vi "Robot.vi"(1 "error in":errorcluster, 2 "Type":enum16{"Mini45", "Simulation", "Joystick"}(ring)=enum."Simulation") -> (0 "error out":errorcluster)   [LabVIEW 2017]
uses:
  <vilib>/Analysis/Matrix/Datatypes/RealMatrix.ctl
  Control/Motor Position.ctl
  Control/Constants.ctl
  Control/Platform Vectors.ctl
  Control/Force Torque Vector.ctl
  Control/RPY.ctl
  <vilib>/Analysis/baseanly.llb/A x Vector.vi
  <vilib>/Analysis/baseanly.llb/Mean (DBL).vi
  <vilib>/Analysis/_algsub.llb/Real Vector Norm.vi
  <vilib>/Analysis/baseanly.llb/Real A x B.vi
  <vilib>/DAQmx/read.llb/DAQmx Read (Analog 2D DBL NChan NSamp).vi
  <vilib>/Analysis/baseanly.llb/Outer Product.vi
  <vilib>/Analysis/baseanly.llb/Real Outer Product.vi
  <vilib>/robotics/Kinematics/Create Lie Group Matrix.vi
  <vilib>/Analysis/7linalg.llb/Create Special Real Matrix.vi
  <vilib>/Analysis/Matrix/Numeric/Multiply/Multiply.vi
  <vilib>/Analysis/Matrix/Numeric/Multiply/Multiply - RM,R.vi
  <vilib>/Analysis/Matrix/Numeric/Multiply/Multiply - R,RM.vi
  <vilib>/Analysis/Matrix/Numeric/Add/Add.vi
  <vilib>/Analysis/Matrix/Numeric/Add/Add - RM,RM.vi
  <vilib>/Analysis/3filter.llb/Butterworth Filter (DBL).vi
  Global.vi
  <vilib>/Utility/inputDevices.llb/joystickAcquire.vi
  <vilib>/DAQmx/create/channels.llb/DAQmx Create Channel (AI-Voltage-Basic).vi
  <vilib>/DAQmx/configure/timing.llb/DAQmx Timing (Sample Clock).vi
  <vilib>/DAQmx/miscellaneous.llb/DAQmx Fill In Error Info.vi
  <vilib>/Analysis/NI_AALBase.lvlib
  <vilib>/robotics/Kinematics/NI_Kinematics.lvlib
  <vilib>/Analysis/NI_AALPro.lvlib
  <vilib>/ptbypt/NI_PtbyPt.lvlib
  <vilib>/Analysis/Matrix/NI_Matrix.lvlib
panel:
  in  "low cutoff freq: fl":dbl=0.1 format="%0.4f"
  in  "sampling freq: fs":dbl=100.0 format="%0.2f"
  in  "rate":dbl=1000.0 format="%#_13g"
  in  "eta3":dbl=240.0
  in  "eta2":dbl=120.0
  in  "eta1":dbl
  in  "gamma2":dbl=72.0
  in  "gamma1":dbl=90.0
  in  "alpha2":dbl=90.0
  in  "alpha1":dbl=90.0
  in  "radius":dbl=0.1
  in  "Calibration Matrix":T1=[[0.70287, 0.28046, -1.06379, -47.58271, -1.64459, 46.90249], [-0.12905, 55.12684, -1.23322, -27.09022, 0.94146, -27.44249], [69.23154, 1.17633, 67.18151, 0.05352, 69.14468, -0.82584], [0.02366, 0.38743, -1.10802, -0.19684, 1.1351, -0.20033], [1.26658, 0.02633, -0.60731, 0.32903, -0.6386, -0.32248], [0.02624, -0.70869, -0.00313, -0.69424, -0.02408, -0.68399]]
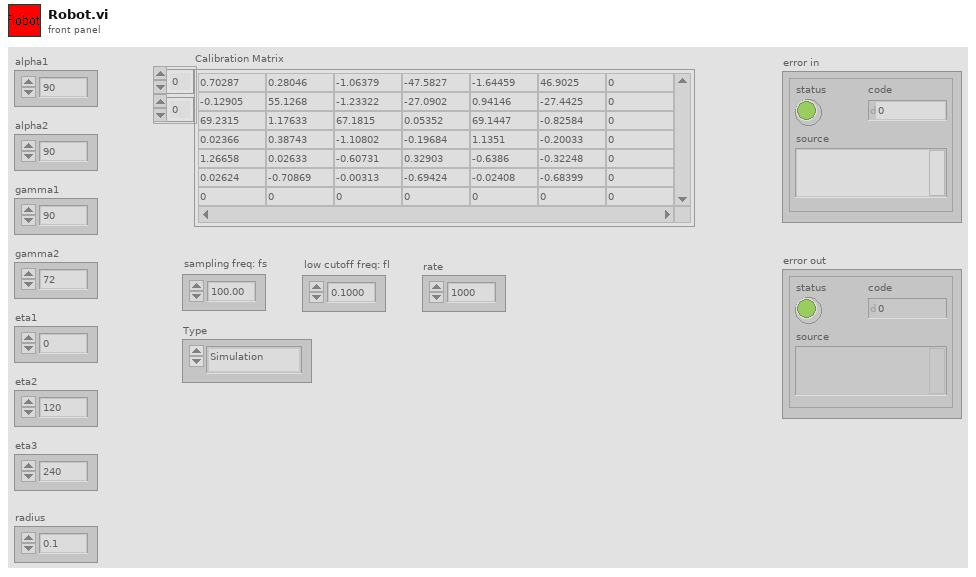
[diagram p1: front panel]
types:
  T1 = typedef "NI_Matrix.lvlib/RealMatrix.ctl" = dbl[][]
  T2 = typedef "Motor Position.ctl" = cluster{"theta1":dbl, "theta2":dbl, "theta3":dbl}
  T3 = typedef "Platform Vectors.ctl" = cluster{"v1":dbl[], "v2":dbl[], "v3":dbl[]}
  T4 = typedef "Constants.ctl" = cluster{"alpha1":dbl, "alpha2":dbl, "beta1":dbl, "beta2":dbl, "gamma1":dbl, "gamma2":dbl, "eta1":dbl, "eta2":dbl, "eta3":dbl}
  T5 = typedef "Force Torque Vector.ctl" = cluster{"Fx":dbl, "Fy":dbl, "Tz":dbl}
  T6 = typedef "RPY.ctl" = cluster{"roll":dbl, "pitch":dbl, "yaw":dbl}
  T7 = cluster{"X axis":i32, "Y axis":i32, "Z axis":i32, "X axis rotation":i32, "Y axis rotation":i32, "Z axis rotation":i32, "U axis":i32, "V axis":i32}
  T8 = typedef "Damping.ctl" = cluster{"Cx":dbl, "Cy":dbl, "Cz":dbl}
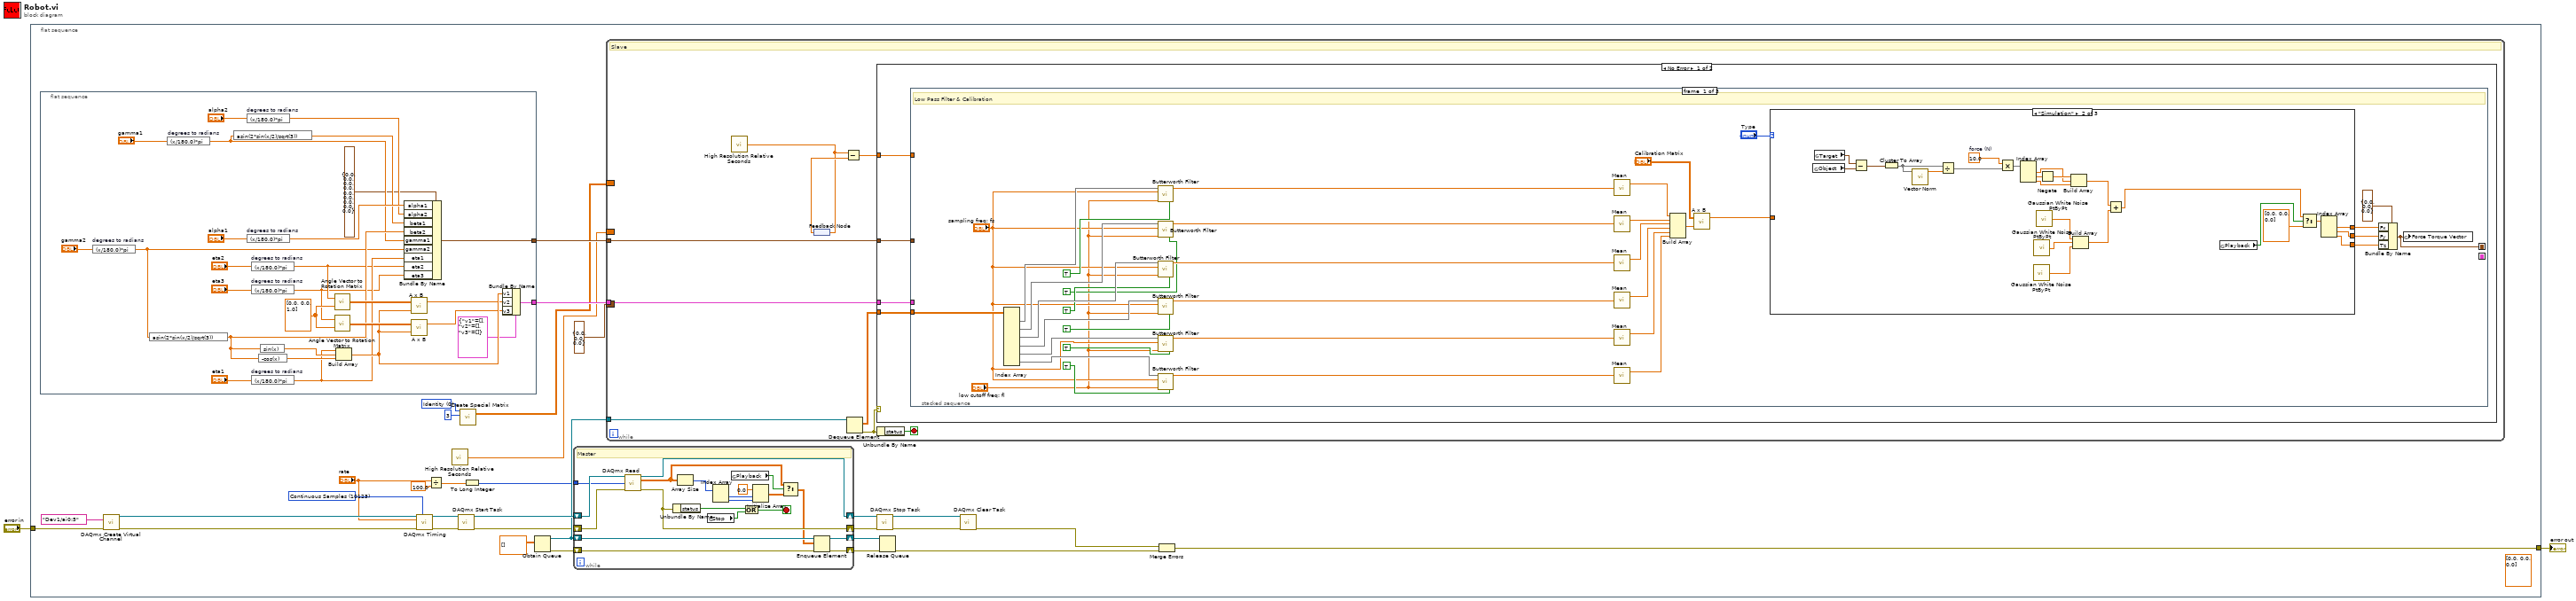
[diagram p0: block diagram]
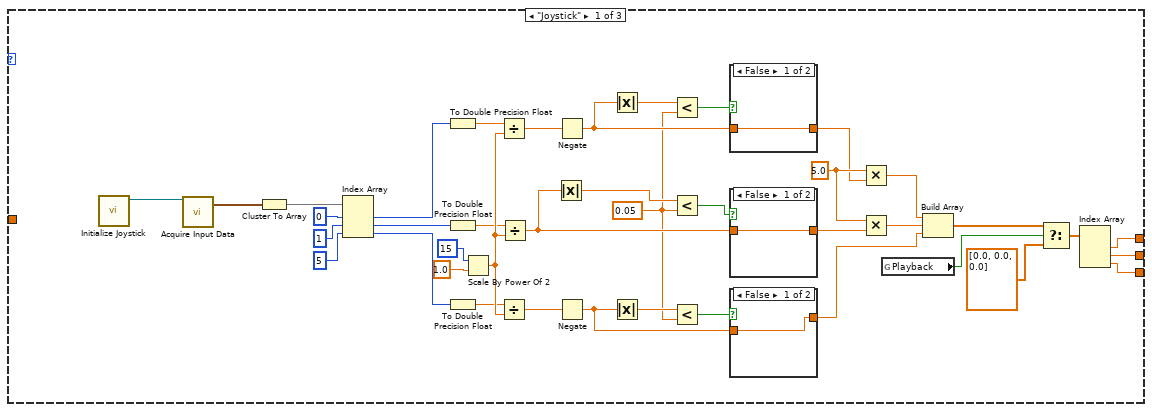
[diagram p2: hidden frame]
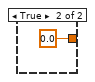
[diagram p3: hidden frame]
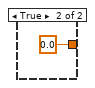
[diagram p4: hidden frame]
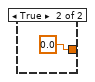
[diagram p5: hidden frame]
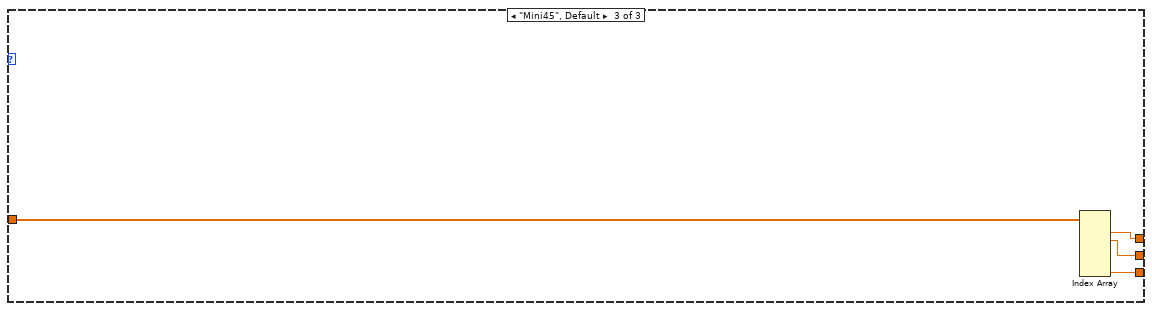
[diagram p6: hidden frame]
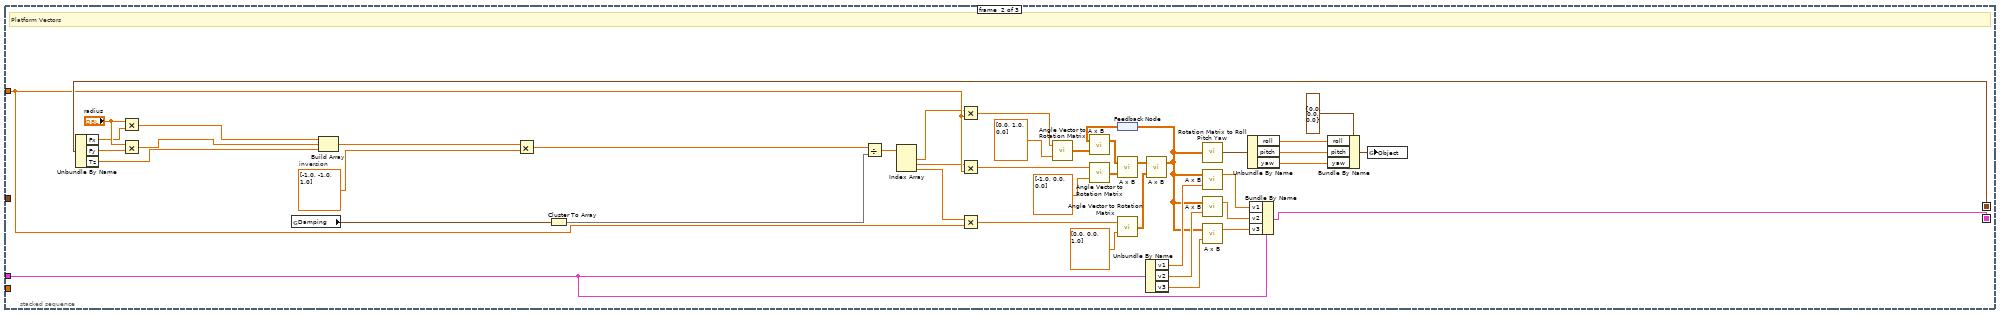
[diagram p7: hidden frame]
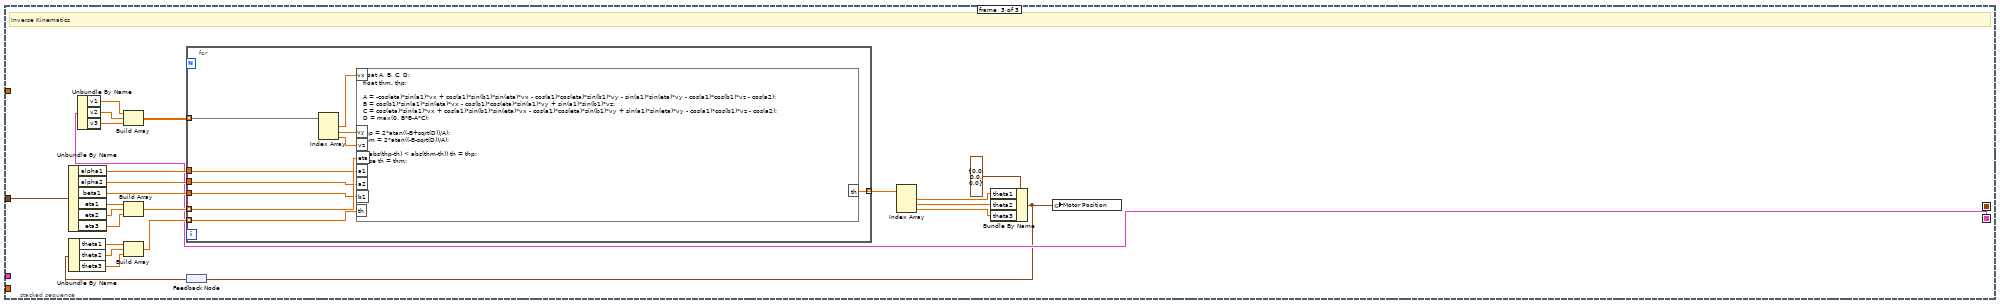
[diagram p8: hidden frame]
diagram:
  n1 = flat-sequence {
    tunnel: "error in" -> [w5]
    tunnel: [w3] -> w1
    frame #0 {
      w16 = 0 items=["Identity", "Diagonal", "Toeplitz", "Vandermonde", "Companion", "Hankel", "Hadamard", "Wilkinson", "Hilbert", "Inverse Hilbert", "Rosser", "Pascal"] ("matrix type")
      (unwired) dbl[] [0.0, 0.0, 0.0]
      w22 = 10123 items=["Finite Samples"=10178, "Continuous Samples"=10123, "Hardware Timed Single Point"=12522] ("sample mode")
      n2 = flat-sequence {
        tunnel: [w62] -> w34
        tunnel: [w61] -> w33
        frame #0 {
          w49 = dbl[] [0.0, 0.0, 1.0] ("vector")
          n3 = expression code="(x/180.0)*pi" "degrees to radians"("gamma2") -> (w43:dbl)
          n4 = expression code="asin(2*sin(x/2)/sqrt(3))"(w43) -> (w45:dbl)
          n5 = expression code="(x/180.0)*pi" "degrees to radians"("gamma1") -> (w44:dbl)
          n6 = expression code="asin(2*sin(x/2)/sqrt(3))"(w44) -> (w56:dbl)
          n7 = expression code="(x/180.0)*pi" "degrees to radians"("alpha2") -> (w57:dbl)
          n8 = expression code="(x/180.0)*pi" "degrees to radians"("alpha1") -> (w59:dbl)
          n9 = expression code="(x/180.0)*pi" "degrees to radians"("eta2") -> (w38:dbl)
          n10 = expression code="(x/180.0)*pi" "degrees to radians"("eta3") -> (w37:dbl)
          n11 = expression code="(x/180.0)*pi" "degrees to radians"("eta1") -> (w39:dbl)
          n12 = expression code="-cos(x)"(w45) -> (w51:dbl)
          n13 = expression code="sin(x)"(w45) -> (w50:dbl)
          n14 = call <vilib>:"Angle Vector to Rotation Matrix.vi"("vector"=w49, "angle"=w38) -> ("rotation matrix"=w52:T1)
          n15 = call <vilib>:"Angle Vector to Rotation Matrix.vi"("vector"=w49, "angle"=w37) -> ("rotation matrix"=w53:T1)
          n16 = Build Array(w39, w50, w51) -> (w48:dbl[])
          n17 = Bundle By Name(cluster=T4 {"alpha1"=0.0, "alpha2"=0.0, "beta1"=0.0, "beta2"=0.0, "gamma1"=0.0, "gamma2"=0.0, "eta1"=0.0, "eta2"=0.0, "eta3"=0.0} ("Constants"), "alpha1"=w59, "alpha2"=w57, "beta1"=w56, "beta2"=w45, "gamma1"=w44, "gamma2"=w43, "eta1"=w39, "eta2"=w38, "eta3"=w37) -> (w61:T4)
          n18 = call-poly <vilib>:"A x B.vi"("Vector"=w48, "A"=w52) -> ("A x Vector"=w47:dbl[])  [unwired: 1 out]
          n19 = call-poly <vilib>:"A x B.vi"("Vector"=w48, "A"=w53) -> ("A x Vector"=w46:dbl[])  [unwired: 1 out]
          n20 = Bundle By Name(cluster=T3 {"v1"=[], "v2"=[], "v3"=[]} ("Platform Vectors"), "v1"=w48, "v2"=w47, "v3"=w46) -> (w62:T3)
        }
      }
      n21 = call-poly <vilib>:"DAQmx Create Virtual Channel.vi"("physical channels"=tag "Dev1/ai0:5", "error in"=w5) -> ("task out"=w31:refnum<k21>, "error out"=w30:errorcluster)  [unwired: 12 in]
      n22 = call-poly <vilib>:"DAQmx Timing.vi"("task/channels in"=w31, "sample mode"=w22, "rate"="rate", "error in"=w30) -> ("task out"=w28:refnum<k21>, "error out"=w29:errorcluster)  [unwired: 10 in]
      n23 = Divide(x="rate", y=100.0) -> (x/y=w6:dbl)
      n24 = call <vilib>:"High Resolution Relative Seconds.vi"() -> ("relative seconds"=w7:dbl)
      n25 = call <vilib>:"DAQmx Start Task.vi"("task/channels in"=w28, "error in"=w29) -> ("task out"=w27:refnum<k21>, "error out"=w4:errorcluster)  [unwired: 12 in]
      n26 = call-poly <vilib>:"Create Special Matrix.vi"("matrix type"=w16, "matrix size"=3) -> ("Special Matrix"=w14:T1)  [unwired: 3 in, 1 out]
      n27 = To Long Integer(number=w6) -> (32bit integer=w9:i32)
      n28 = Obtain Queue(element data type=dbl[][] [] ("data")) -> (queue out=w12:refnum<queue>, error out=w21:errorcluster)  [unwired: 4 in, 1 out]
      n29 = while {
        shift-right: [w278] -> w19
        shift-left: w12 -> [w279]
        shift-right: [w275] -> w18
        shift-left: w21 -> [w277]
        shift-right: [w282] -> w26
        shift-left: w27 -> [w283]
        shift-right: [w280] -> w24
        shift-left: w4 -> [w281]
        tunnel: w9 -> [w273]
        stop <- w274 stop-if-true
        # "Master"
        n30 = call-poly <vilib>:"DAQmx Read.vi"("task/channels in"=w283, "number of samples per channel"=w273, "error in"=w281) -> ("task out"=w282:refnum<k21>, "data"=w269:dbl[][], "error out"=w280:errorcluster)  [unwired: 10 in]
        n31 = Unbundle By Name(w280) -> ("status"=w276:bool)
        n32 = Array Size(array=w269) -> (size(s)=w268:i32[])
        n33 = global read "Global.vi" "Stop"() -> (w272:bool)
        n34 = Index Array(array=w268) -> (element #1=w267:i32, element #2=w266:i32)  [unwired: 2 in]
        n35 = global read "Global.vi" "Playback"() -> (w271:bool)
        n36 = Compound Arithmetic op=OR(w276, w272) -> (w274:bool)
        n37 = Initialize Array(0.0 ("element"), w267, w266) -> (w264:dbl[][])
        n38 = Select(t=w269, s=w271, f=w264) -> (s? t:f=w270:dbl[][])
        n39 = Enqueue Element(queue=w279, element=w270, error in (no error)=w277) -> (queue out=w278:refnum<queue>, error out=w275:errorcluster)  [unwired: 1 in, 1 out]
      }
      n40 = while {
        tunnel: w12 -> [w71]
        border: w14 -> [_]
        tunnel: w33 -> [w69]
        border: T2 {"theta1"=0.0, "theta2"=0.0, "theta3"=0.0} ("Motor Position") -> [_]
        border: w7 -> [_]
        tunnel: w34 -> [w70]
        stop <- w63 stop-if-true
        # "Slave"
        n41 = call <vilib>:"High Resolution Relative Seconds.vi"() -> ("relative seconds"=w65:dbl)
        n42 = feedback-in #1(w65) -> ()
        n43 = feedback #1() -> (w66:dbl)
        n44 = Subtract(x=w65, y=w66) -> (x-y=w64:dbl)
        n45 = Dequeue Element(queue=w71) -> (element=w67:dbl[][], error out=w68:errorcluster)  [unwired: 2 in, 2 out]
        n46 = case shown="No Error" w68 {
          tunnel: w70 -> [w75 _]
          tunnel: w69 -> [w74 _]
          tunnel: w67 -> [w73 _]
          tunnel: w64 -> [w72 _]
          frame No Error {
            n47 = stacked-sequence {
              seq-local: [w76 _ _] -> [_ w219 _]
              seq-local: [_ w205 _] -> [_ _ w232]
              tunnel: w75 -> [_ w208 _]
              tunnel: w74 -> [_ _ w249]
              tunnel: w72 -> [_ w204 _]
              tunnel: w73 -> [w87 _ _]
              frame #0 {
                # "Low Pass Filter & Calibration"
                n48 = Index Array(array=w87) -> (element #1=w98:dbl[], element #2=w97:dbl[], element #3=w96:dbl[], element #4=w95:dbl[], element #5=w94:dbl[], element #6=w93:dbl[])  [unwired: 12 in]
                n49 = call-poly <vilib>:"Butterworth Filter.vi"("init/cont (init:F)"=TRUE, "low cutoff freq: fl"="low cutoff freq: fl", "sampling freq: fs"="sampling freq: fs", "X"=w98) -> ("Filtered X"=w99:dbl[])  [unwired: 4 in, 1 out]
                n50 = call-poly <vilib>:"Butterworth Filter.vi"("init/cont (init:F)"=TRUE, "low cutoff freq: fl"="low cutoff freq: fl", "sampling freq: fs"="sampling freq: fs", "X"=w97) -> ("Filtered X"=w101:dbl[])  [unwired: 4 in, 1 out]
                n51 = call-poly <vilib>:"Butterworth Filter.vi"("init/cont (init:F)"=TRUE, "low cutoff freq: fl"="low cutoff freq: fl", "sampling freq: fs"="sampling freq: fs", "X"=w96) -> ("Filtered X"=w103:dbl[])  [unwired: 4 in, 1 out]
                n52 = call-poly <vilib>:"Butterworth Filter.vi"("init/cont (init:F)"=TRUE, "low cutoff freq: fl"="low cutoff freq: fl", "sampling freq: fs"="sampling freq: fs", "X"=w95) -> ("Filtered X"=w104:dbl[])  [unwired: 4 in, 1 out]
                n53 = call-poly <vilib>:"Butterworth Filter.vi"("init/cont (init:F)"=TRUE, "low cutoff freq: fl"="low cutoff freq: fl", "sampling freq: fs"="sampling freq: fs", "X"=w94) -> ("Filtered X"=w105:dbl[])  [unwired: 4 in, 1 out]
                n54 = call-poly <vilib>:"Butterworth Filter.vi"("init/cont (init:F)"=TRUE, "low cutoff freq: fl"="low cutoff freq: fl", "sampling freq: fs"="sampling freq: fs", "X"=w93) -> ("Filtered X"=w109:dbl[])  [unwired: 4 in, 1 out]
                n55 = call-poly <vilib>:"Mean.vi"("X"=w99) -> ("mean"=w100:dbl)  [unwired: 1 out]
                n56 = call-poly <vilib>:"Mean.vi"("X"=w101) -> ("mean"=w102:dbl)  [unwired: 1 out]
                n57 = call-poly <vilib>:"Mean.vi"("X"=w103) -> ("mean"=w106:dbl)  [unwired: 1 out]
                n58 = call-poly <vilib>:"Mean.vi"("X"=w104) -> ("mean"=w107:dbl)  [unwired: 1 out]
                n59 = call-poly <vilib>:"Mean.vi"("X"=w105) -> ("mean"=w108:dbl)  [unwired: 1 out]
                n60 = call-poly <vilib>:"Mean.vi"("X"=w109) -> ("mean"=w110:dbl)  [unwired: 1 out]
                n61 = Build Array(w100, w102, w106, w107, w108, w110) -> (w85:dbl[])
                n62 = call-poly <vilib>:"A x B.vi"("Vector"=w85, "A"="Calibration Matrix") -> ("A x Vector"=w81:dbl[])  [unwired: 1 out]
                n63 = case shown="\"Simulation\"" "Type" {
                  tunnel: w81 -> [_ _ w185]
                  tunnel: [w115 w181 w184] -> w79
                  tunnel: [w114 w180 w183] -> w78
                  tunnel: [w113 w179 w182] -> w77
                  frame "Joystick" {
                    w124 = 5.0 ("element")
                    w131 = 0.05 ("y")
                    n64 = call <vilib>:"Initialize Joystick.vi"() -> ("device ID"=w144:refnum<k1>)  [unwired: 10 in, 1 out]
                    n65 = call-poly <vilib>:"Acquire Input Data.vi"("device ID"=w144) -> ("axis info"=w151:T7)  [unwired: 14 in, 4 out]
                    n66 = Cluster To Array(cluster=w151) -> (array=w147:i32[])
                    n67 = Index Array(array=w147, index #1=0 ("index"), index #2=1 ("index"), index #3=5 ("index")) -> (element #1=w130:i32, element #2=w128:i32, element #3=w126:i32)
                    n68 = To Double Precision Float(number=w130) -> (double precision float=w129:dbl)
                    n69 = To Double Precision Float(number=w128) -> (double precision float=w127:dbl)
                    n70 = To Double Precision Float(number=w126) -> (double precision float=w125:dbl)
                    n71 = Scale By Power Of 2(n=i16 15, x=1.0) -> (x*2^n=w139:dbl)
                    n72 = Divide(x=w129, y=w139) -> (x/y=w143:dbl)
                    n73 = Divide(x=w125, y=w139) -> (x/y=w132:dbl)
                    n74 = Divide(x=w127, y=w139) -> (x/y=w134:dbl)
                    n75 = Absolute Value(x=w134) -> (abs(x)=w141:dbl)
                    n76 = Negate(x=w143) -> (-x=w135:dbl)
                    n77 = Negate(x=w132) -> (-x=w133:dbl)
                    n78 = Absolute Value(x=w135) -> (abs(x)=w142:dbl)
                    n79 = Absolute Value(x=w133) -> (abs(x)=w140:dbl)
                    n80 = Less?(x=w142, y=w131) -> (x < y?=w138:bool)
                    n81 = Less?(x=w141, y=w131) -> (x < y?=w137:bool)
                    n82 = Less?(x=w140, y=w131) -> (x < y?=w136:bool)
                    n83 = case shown="False" w138 {
                      tunnel: [w156 0.0] -> w123
                      tunnel: w135 -> [w156 _]
                      frame False {
                      }
                      frame True {
                      }
                    }
                    n84 = case shown="False" w137 {
                      tunnel: [w154 0.0] -> w122
                      tunnel: w134 -> [w154 _]
                      frame False {
                      }
                      frame True {
                      }
                    }
                    n85 = case shown="False" w136 {
                      tunnel: [w152 0.0] -> w118
                      tunnel: w133 -> [w152 _]
                      frame False {
                      }
                      frame True {
                      }
                    }
                    n86 = Multiply(x=w124, y=w123) -> (x*y=w120:dbl)
                    n87 = Multiply(x=w124, y=w122) -> (x*y=w119:dbl)
                    n88 = global read "Global.vi" "Playback"() -> (w121:bool)
                    n89 = Build Array(w120, w119, w118) -> (w117:dbl[])
                    n90 = Select(t=w117, s=w121, f=dbl[] [0.0, 0.0, 0.0]) -> (s? t:f=w116:dbl[])
                    n91 = Index Array(array=w116) -> (element #1=w115:dbl, element #2=w114:dbl, element #3=w113:dbl)  [unwired: 3 in]
                  }
                  frame "Simulation" {
                    w171 = 10.0  # force (N)
                    n92 = global read "Global.vi" "Object"() -> (w169:T6)
                    n93 = global read "Global.vi" "Target"() -> (w170:T6)
                    n94 = Subtract(x=w170, y=w169) -> (x-y=w175:T6)
                    n95 = Cluster To Array(cluster=w175) -> (array=w174:dbl[])
                    n96 = call-poly <vilib>:"Vector Norm.vi"("Input Vector"=w174) -> ("norm"=w173:dbl)  [unwired: 9 in, 1 out]
                    n97 = Divide(x=w174, y=w173) -> (x/y=w172:dbl[])
                    n98 = Multiply(x=w171, y=w172) -> (x*y=w166:dbl[])
                    n99 = Index Array(array=w166) -> (element #1=w165:dbl, element #2=w168:dbl, element #3=w164:dbl)  [unwired: 3 in]
                    n100 = call <vilib>:"Gaussian White Noise PtByPt.vi"() -> ("Gaussian white noise"=w161:dbl)  [unwired: 3 in]
                    n101 = call <vilib>:"Gaussian White Noise PtByPt.vi"() -> ("Gaussian white noise"=w162:dbl)  [unwired: 3 in]
                    n102 = call <vilib>:"Gaussian White Noise PtByPt.vi"() -> ("Gaussian white noise"=w163:dbl)  [unwired: 3 in]
                    n103 = Negate(x=w168) -> (-x=w167:dbl)
                    n104 = Build Array(w167, w165, w164) -> (w160:dbl[])
                    n105 = Build Array(w163, w162, w161) -> (w159:dbl[])
                    n106 = Add(x=w160, y=w159) -> (x+y=w158:dbl[])
                    n107 = global read "Global.vi" "Playback"() -> (w176:bool)
                    n108 = Select(t=w158, s=w176, f=dbl[] [0.0, 0.0, 0.0]) -> (s? t:f=w178:dbl[])
                    n109 = Index Array(array=w178) -> (element #1=w181:dbl, element #2=w180:dbl, element #3=w179:dbl)  [unwired: 3 in]
                  }
                  frame "Mini45", Default {
                    n110 = Index Array(array=w185) -> (element #1=w184:dbl, element #2=w183:dbl, element #6=w182:dbl)  [unwired: 6 in, 3 out]
                  }
                }
                n111 = Bundle By Name(cluster=T5 {"Fx"=0.0, "Fy"=0.0, "Tz"=0.0} ("Force Torque Vector"), "Fx"=w79, "Fy"=w78, "Tz"=w77) -> (w76:T5)
                n112 = global write "Global.vi" "Force Torque Vector"(w76) -> ()
              }
              frame #1 {
                w206 = dbl[] [-1.0, -1.0, 1.0]  # inversion
                # "Platform Vectors"
                n113 = Unbundle By Name(w219) -> ("Fx"=w217:dbl, "Fy"=w216:dbl, "Tz"=w213:dbl)
                n114 = Multiply(x="radius", y=w217) -> (x*y=w215:dbl)
                n115 = Multiply(x="radius", y=w216) -> (x*y=w214:dbl)
                n116 = global read "Global.vi" "Damping"() -> (w191:T8)
                n117 = Build Array(w215, w214, w213) -> (w207:dbl[])
                n118 = Multiply(x=w207, y=w206) -> (x*y=w192:dbl[])
                n119 = Cluster To Array(cluster=w191) -> (array=w190:dbl[])
                n120 = Divide(x=w192, y=w190) -> (x/y=w189:dbl[])
                n121 = Index Array(array=w189) -> (element #1=w188:dbl, element #2=w187:dbl, element #3=w186:dbl)  [unwired: 3 in]
                n122 = Multiply(x=w188, y=w204) -> (x*y=w229:dbl)
                n123 = Multiply(x=w187, y=w204) -> (x*y=w228:dbl)
                n124 = Multiply(x=w186, y=w204) -> (x*y=w203:dbl)
                n125 = call <vilib>:"Angle Vector to Rotation Matrix.vi"("vector"=dbl[] [0.0, 1.0, 0.0], "angle"=w229) -> ("rotation matrix"=w224:T1)
                n126 = call <vilib>:"Angle Vector to Rotation Matrix.vi"("vector"=dbl[] [-1.0, 0.0, 0.0], "angle"=w228) -> ("rotation matrix"=w222:T1)
                n127 = feedback #2() -> (w212:T1)
                n128 = call-poly <vilib>:"A x B.vi"("B"=w224, "A"=w212) -> ("A x B"=w223:T1)  [unwired: 1 out]
                n129 = call-poly <vilib>:"A x B.vi"("B"=w222, "A"=w223) -> ("A x B"=w221:T1)  [unwired: 1 out]
                n130 = call <vilib>:"Angle Vector to Rotation Matrix.vi"("vector"=dbl[] [0.0, 0.0, 1.0], "angle"=w203) -> ("rotation matrix"=w220:T1)
                n131 = Unbundle By Name(w208) -> ("v1"=w211:dbl[], "v2"=w210:dbl[], "v3"=w209:dbl[])
                n132 = call-poly <vilib>:"A x B.vi"("B"=w220, "A"=w221) -> ("A x B"=w199:T1)  [unwired: 1 out]
                n133 = feedback-in #2(w199) -> ()
                n134 = call <vilib>:"Rotation Matrix to Roll Pitch Yaw.vi"("rotation matrix"=w199) -> ("angles"=w197:cluster{"roll":dbl, "pitch":dbl, "yaw":dbl})
                n135 = call-poly <vilib>:"A x B.vi"("Vector"=w211, "A"=w199) -> ("A x Vector"=w202:dbl[])  [unwired: 1 out]
                n136 = call-poly <vilib>:"A x B.vi"("Vector"=w210, "A"=w199) -> ("A x Vector"=w201:dbl[])  [unwired: 1 out]
                n137 = call-poly <vilib>:"A x B.vi"("Vector"=w209, "A"=w199) -> ("A x Vector"=w200:dbl[])  [unwired: 1 out]
                n138 = Unbundle By Name(w197) -> ("roll"=w196:dbl, "pitch"=w195:dbl, "yaw"=w194:dbl)
                n139 = Bundle By Name(cluster=w208, "v1"=w202, "v2"=w201, "v3"=w200) -> (w205:T3)
                n140 = Bundle By Name(cluster=T6 {"roll"=0.0, "pitch"=0.0, "yaw"=0.0} ("RPY"), "roll"=w196, "pitch"=w195, "yaw"=w194) -> (w193:T6)
                n141 = global write "Global.vi" "Object"(w193) -> ()
              }
              frame #2 {
                # "Inverse Kinematics"
                n142 = Unbundle By Name(w249) -> ("alpha1"=w244:dbl, "alpha2"=w243:dbl, "beta1"=w242:dbl, "eta1"=w248:dbl, "eta2"=w247:dbl, "eta3"=w246:dbl)
                n143 = Unbundle By Name(w232) -> ("v1"=w253:dbl[], "v2"=w252:dbl[], "v3"=w251:dbl[])
                n144 = Build Array(w253, w252, w251) -> (w250:dbl[][])
                n145 = Build Array(w248, w247, w246) -> (w245:dbl[])
                n146 = feedback #3() -> (w237:T2)
                n147 = Unbundle By Name(w237) -> ("theta1"=w236:dbl, "theta2"=w235:dbl, "theta3"=w234:dbl)
                n148 = Build Array(w236, w235, w234) -> (w233:dbl[])
                n149 = for {
                  tunnel: w250 -> [w263] mode=indexing
                  tunnel: w245 -> [w259] mode=indexing
                  tunnel: w244 -> [w258]
                  tunnel: w243 -> [w257]
                  tunnel: w242 -> [w256]
                  tunnel: [w255] -> w241 mode=indexing
                  tunnel: w233 -> [w254] mode=indexing
                  n150 = Index Array(array=w263) -> (element #1=w262:dbl, element #2=w261:dbl, element #3=w260:dbl)  [unwired: 3 in]
                  n151 = formula code="float A, B, C, D;\nfloat thm, thp;\n\nA = -cos(eta)*sin(a1)*vx + cos(a1)*sin(b1)*sin(eta)*vx - cos(a1)*cos(eta)*sin(b1)*vy - sin(a1)*sin(eta)*vy - cos(a1)*cos(b1)*vz - cos(a2);\nB = cos(b1)*sin(a1)*sin(eta)*vx - cos(b1)*cos(eta)*sin(a1)*vy + sin(a1)*sin(b1)*vz;\nC = cos(eta)*sin(a1)*vx + cos(a1)*sin(b1)*sin(eta)*vx - cos(a1)*cos(eta)*sin(b1)*vy + sin(a1)*sin(eta)*vy - cos(a1)*cos(b1)*vz - cos(a2);\nD = max(0, B*B-A*C);\n\nthp = 2*atan((-B+sqrt(D))/A); \nthm = 2*atan((-B-sqrt(D))/A); \n\nif(abs(thp-th) < abs(thm-th)) th = thp;\nelse th = thm;"("vx"=w262, "vy"=w261, "vz"=w260, "eta"=w259, "a1"=w258, "b1"=w256, "a2"=w257, "th"=w254) -> ("th"=w255:dbl)
                }
                n152 = Index Array(array=w241) -> (element #1=w240:dbl, element #2=w239:dbl, element #3=w238:dbl)  [unwired: 3 in]
                n153 = Bundle By Name(cluster=T2 {"theta1"=0.0, "theta2"=0.0, "theta3"=0.0} ("Motor Position"), "theta1"=w240, "theta2"=w239, "theta3"=w238) -> (w230:T2)
                n154 = feedback-in #3(w230) -> ()
                n155 = global write "Global.vi" "Motor Position"(w230) -> ()
              }
            }
          }
          frame Error {
          }
        }
        n156 = Unbundle By Name(w68) -> ("status"=w63:bool)
      }
      n157 = call <vilib>:"DAQmx Stop Task.vi"("task/channels in"=w26, "error in"=w24) -> ("task out"=w25:refnum<k21>, "error out"=w23:errorcluster)  [unwired: 12 in]
      n158 = Release Queue(queue=w19, error in (no error)=w18) -> (error out=w17:errorcluster)  [unwired: 1 in, 2 out]
      n159 = call <vilib>:"DAQmx Clear Task.vi"("task in"=w25, "error in"=w23) -> ("error out"=w20:errorcluster)  [unwired: 13 in]
      n160 = Merge Errors(w20, w17) -> (w3:errorcluster)
    }
  }
  "error out" <- w1
